vi "One 8-bit Port Digital Output.vi"(2 "Packet":u64, 4 "8-Bit DO Port":refnum<k21>="Chassis1/Mod3/DO7:0") -> ()   [LabVIEW 2010]
uses:
  <vilib>/eio/EIONode/EIONode.xnode
  <vilib>/rvi/eio/nirviEIOImplementation/nirviEIOImplementation.xnode
  <vilib>/rvi/eio/common/nirviEmuClasses.ctl
  <vilib>/rvi/eio/common/nirviEmuTemplateMethod_noerrors.vi
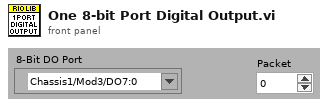
[diagram p1: front panel]
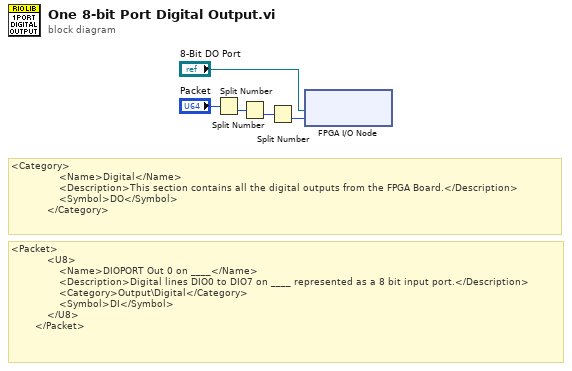
[diagram p0: block diagram]
diagram:
  # "<Packet>\n            <U8>\n                <Name>DIOPORT Out 0 on ____</Name>\n                <Description>Digital lines DIO0 to DIO7 on ____ represented as a 8 bit input port.</Description>\n                <Category>Output\\Digital</Category>\n                <Symbol>DI</Symbol>\n            </U8>\n        </Packet>"
  # "<Category>\n                <Name>Digital</Name>\n                <Description>This section contains all the digital outputs from the FPGA Board.</Description>\n                <Symbol>DO</Symbol>\n            </Category>"
  n1 = Split Number(x="Packet") -> (lo(x)=w4:u32)  [unwired: 1 out]
  n2 = Split Number(x=w4) -> (lo(x)=w5:u16)  [unwired: 1 out]
  n3 = Split Number(x=w5) -> (lo(x)=w2:u8)  [unwired: 1 out]
  n4 = xnode "FPGA I/O Node"("I/O Item"=w2, "FPGA I/O In"="8-Bit DO Port") -> ()  [unwired: 1 out]
